vi "Manual Assembly DB.vi"() -> ()   [LabVIEW 2021]
uses:
  Classes/Routine/Routine Enum.ctl
  Classes/Assembly/Database Entry/Database Entry.lvclass
  Classes/Assembly/Assembly Run.lvclass
  Classes/Workspace/Fixture Enum.ctl
  <vilib>/Utility/file.llb/Read Delimited Spreadsheet (string).vi
  SubVIs/PUT_region.vi
  SubVIs/component_tray_region.vi
  SubVIs/assembly_tray_region.vi
  Classes/Controller/I-O/I-O.lvclass
  Classes/Routine/Routine.lvclass
  Classes/Workspace/Fixture.lvclass
  Classes/Controller/Controller.lvclass
panel:
  out "Dummy assembly":bool
  in  "Do old-style single-module data-entry?":bool
  in  "Update comments":bool
  out "Status":string
  out "Stack names":T1
  out "Feet check":bool
  out "Assembly Type":string
  out "Assembly tray region":dbl
  out "Component tray region":dbl
  out "PUT Region":dbl
  in  "Clear All":bool
  in  "Assemble":bool
  in  "Pick and Place":bool
  in  "Dispense glue":bool
  in  "Go":bool
  in  "Routine":T2=enum."Dispense Epoxy"
  in  "Update":bool
  in  "Stage":i32(listbox)=-1
  in  "Stop":bool
  in  "Remove":bool
  in  "Add":bool
  # "Click the Run arrow to start\nFill out pop-up prompts\nSelect Full Assemble\nSelect GO"
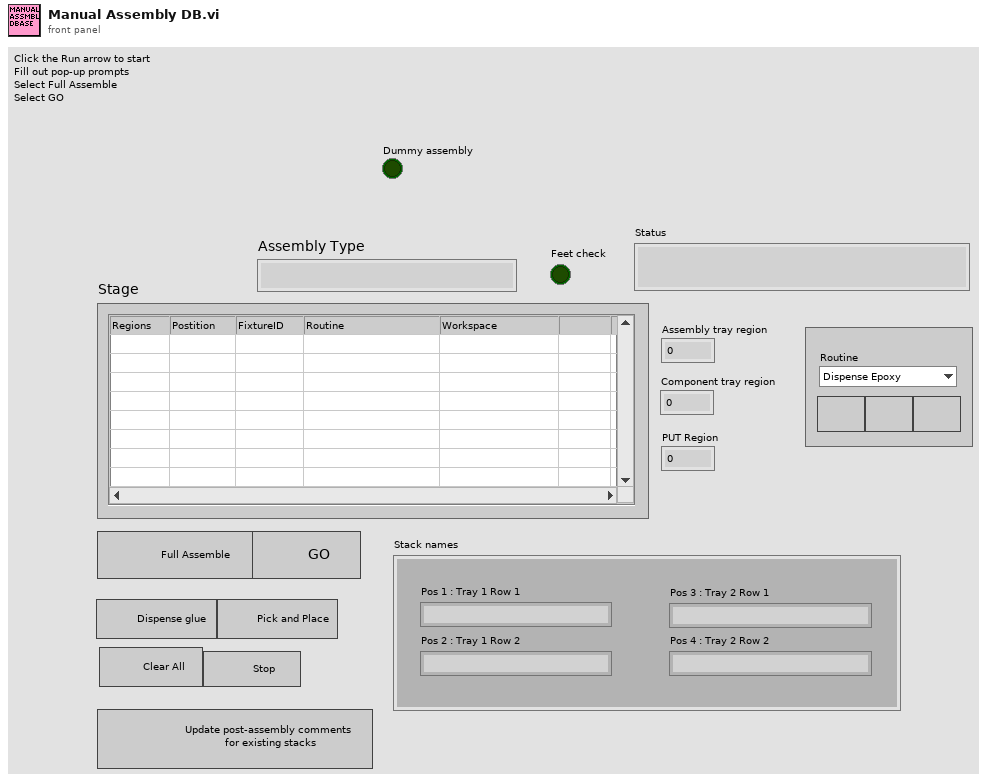
[diagram p1: front panel]
types:
  T1 = cluster{"Pos 1 : Tray 1 Row 1":string, "Pos 2 : Tray 1 Row 2":string, "Pos 3 : Tray 2 Row 1":string, "Pos 4 : Tray 2 Row 2":string}
  T2 = typedef "Routine.lvclass/Routine Enum.ctl" = enum16{"Primary Pick Up", "Secondary Pick Up", "Put Down All", "Secure Syringe", "Release Syringe", "Dispense Epoxy", "Pick Up All", "Put Down Secondary", "Full Assembly"}
  T3 = enum8{"Enabled", "Disabled", "Disabled and Grayed Out"}
  T4 = typedef "Fixture.lvclass/Fixture Enum.ctl" = enum16{"Assembly Tray", "Syringe Space", "Component", "Pick Up Tool", "Current Position"}
  T5 = cluster{"Fixture ID":dbl, "Position":dbl, "Thickness":dbl}
  T6 = typedef "File Paths.ctl" = cluster{"Glue Pattern Folder":path, "Carrier Tray Folder":path, "Pick Up Tool Fixture Folder":path, "Components Folder":path, "Bellows Tool Offset.txt":path, "Pick Up Tool Offset.txt":path, "Dispense Tip Offset.txt":path, "Log Files":path, "Gantry Assembly Map.txt":path, "Syringe and offset map.txt":path, "Controllers Folder":path, "Local dbase config":path}
  T7 = typedef "Controller.lvclass/Controllers.ctl" = cluster{"I-O.lvclass":refnum<class "I-O.lvclass">, "Gantry":refnum<k24>, "Dispenser":refnum<visa-resource-name>}
  T8 = cluster{"Fixture ID":dbl, "Position":dbl, "Thickness":dbl}[]
  T9 = cluster{"Stack names[0]":string, "Stack names[1]":string, "Stack names[2]":string, "Stack names[3]":string}
  T10 = cluster{"Fixture ID":dbl, "Position":dbl, "Thickness":dbl}[][]
  T11 = typedef "I-O.lvclass/Pin Map.ctl" = cluster{"Region Valves":i32[], "Extra Valves":dbl[][][], "Tool Primary Valve":i32, "Tool Secondary Valve":i32, "Region Sensors":i32[], "Extra Sensors":dbl[][][], "Tool Primary Sensor":dbl, "Tool Secondary Sensor":dbl, "Compression Sensor":dbl, "5V":i32, "Dispenser Sensor":dbl}
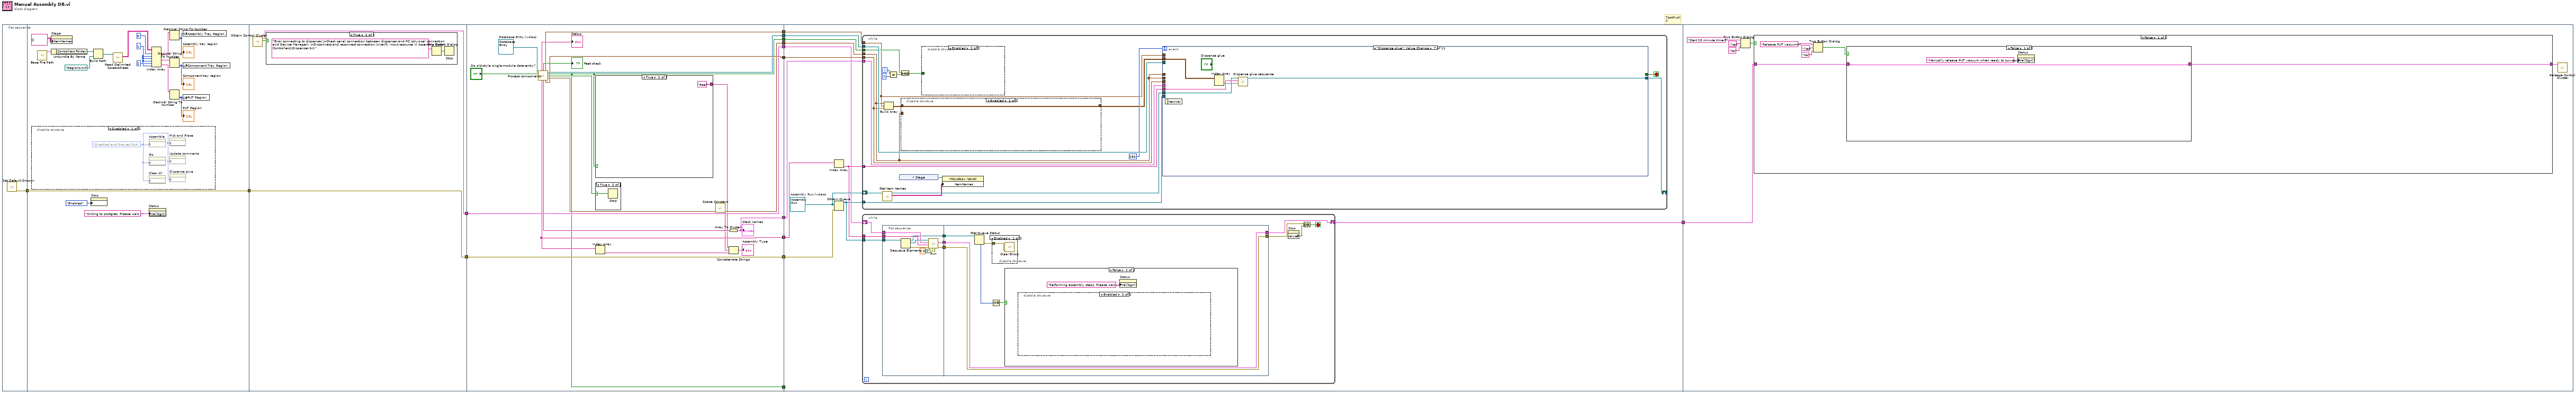
[diagram p0: block diagram]
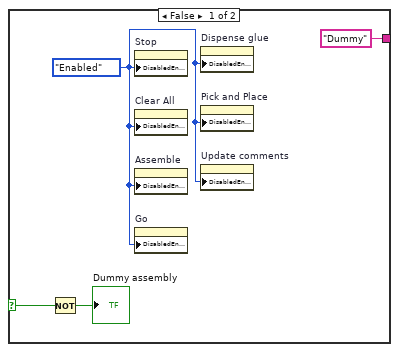
[diagram p4: hidden frame]
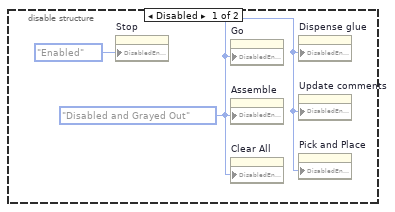
[diagram p7: hidden frame]
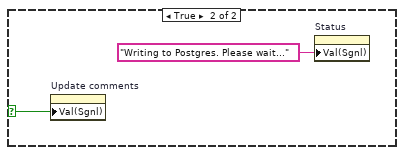
[diagram p8: hidden frame]
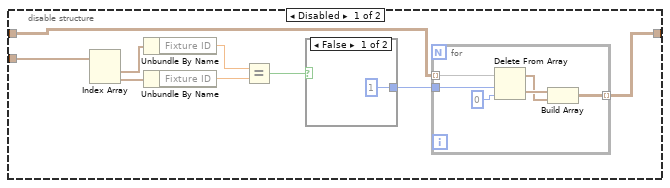
[diagram p9: hidden frame]
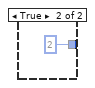
[diagram p10: hidden frame]
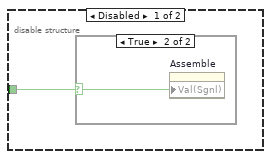
[diagram p11: hidden frame]
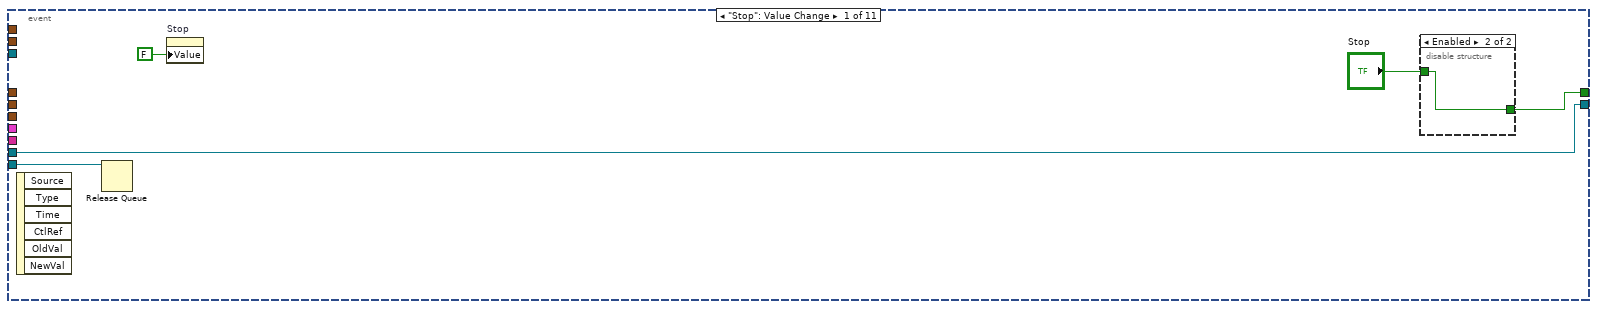
[diagram p13: hidden frame]
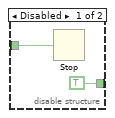
[diagram p14: hidden frame]
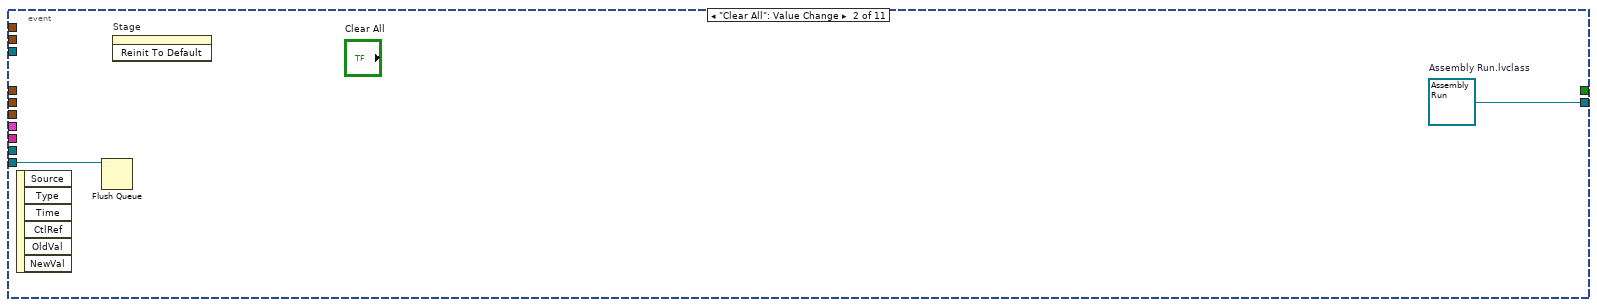
[diagram p15: hidden frame]
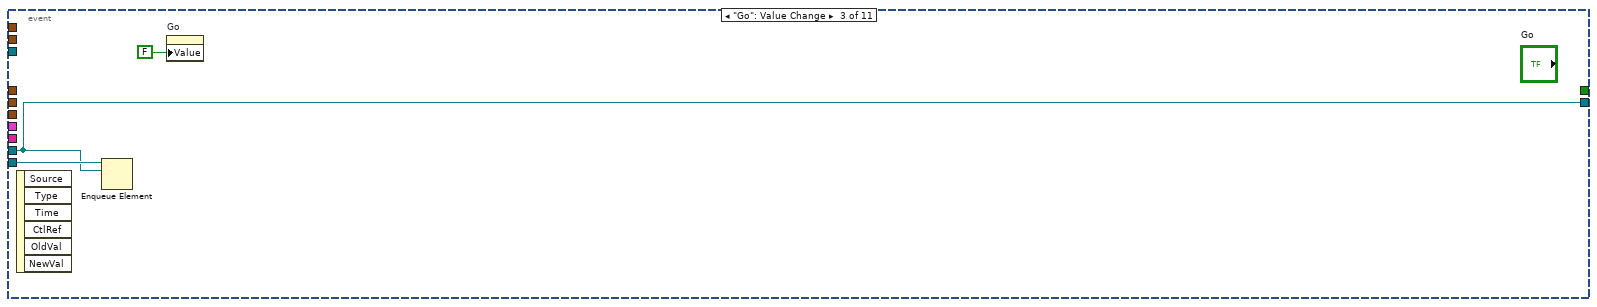
[diagram p16: hidden frame]
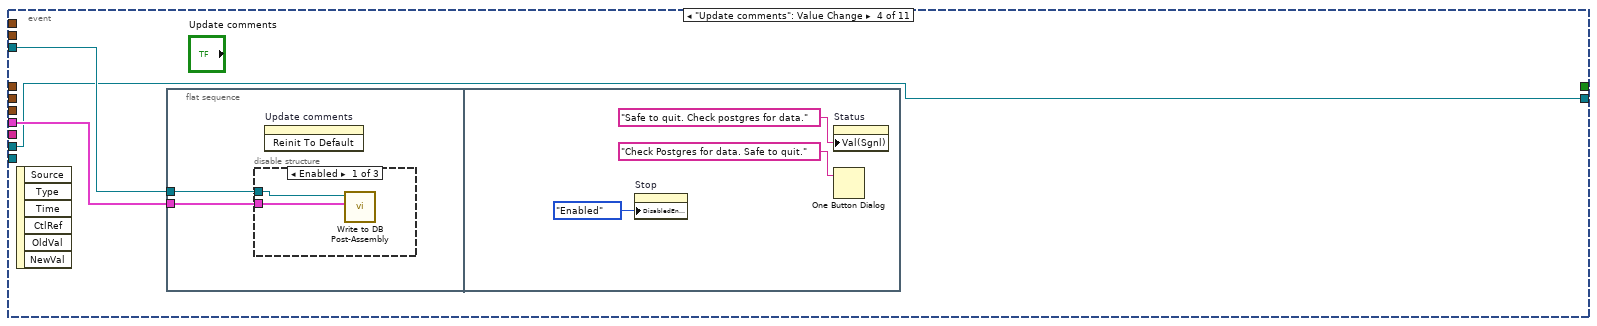
[diagram p17: hidden frame]
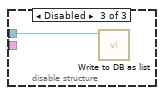
[diagram p19: hidden frame]
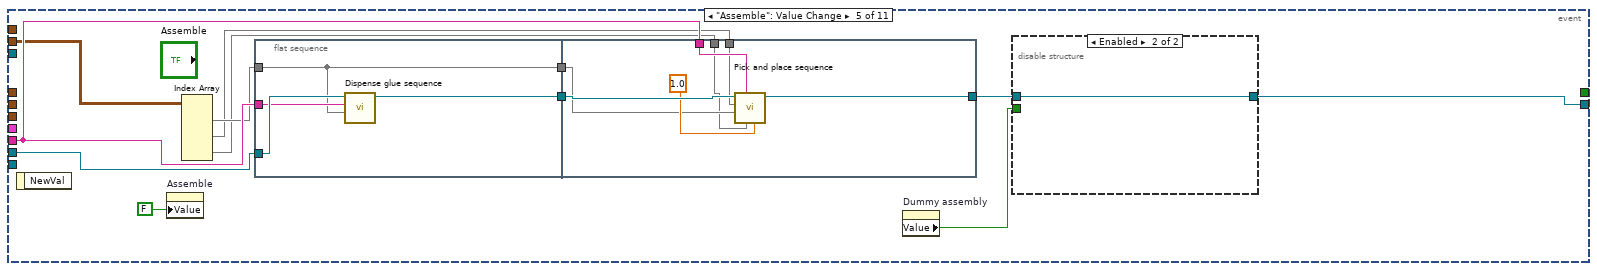
[diagram p20: hidden frame]
diagram:
  # "TestPush\n2"
  n1 = flat-sequence {
    tunnel: [w16] -> w14
    tunnel: [w20] -> w7
    tunnel: w14 -> [w20]
    tunnel: w7 -> [w38]
    tunnel: [w38] -> w6
    tunnel: [w36] -> w4
    tunnel: [w58] -> w15
    tunnel: w6 -> [w58]
    tunnel: [w57] -> w13
    tunnel: [w56] -> w12
    tunnel: [w55] -> w11
    tunnel: [w47] -> w10
    tunnel: [w51] -> w9
    tunnel: [w49] -> w8
    tunnel: [w42] -> w5
    tunnel: w4 -> [w42]
    tunnel: [w41] -> w3
    tunnel: [w41] -> w2
    tunnel: w15 -> [w77]
    tunnel: w13 -> [w76]
    tunnel: w12 -> [w75]
    tunnel: w11 -> [w69]
    tunnel: w10 -> [w74]
    tunnel: w9 -> [w71]
    tunnel: w8 -> [w72]
    tunnel: w5 -> [w68]
    tunnel: w3 -> [w67]
    tunnel: w2 -> [_]
    tunnel: [w66] -> w1
    tunnel: w1 -> [w370]
    frame #0 {
      n2 = call "Set Default Drop-In.vi"() -> ("error out"=w16:errorcluster)  [unwired: 11 in]
    }
    frame #1 {
      w23 = 1 ("disabled index (col)")
      n3 = disable-structure shown="Disabled" {
        frame Disabled {
          w35 = T3."Disabled and Grayed Out" ("Disabled")
          n4 = property on="Assemble" class="Bool (strict)"("DisabledEnum"=w35) -> ()  [unwired: 2 in, 2 out]
          n5 = property on="Go" class="Bool (strict)"("DisabledEnum"=w35) -> ()  [unwired: 2 in, 2 out]
          n6 = property on="Clear All" class="Bool"("DisabledEnum"=w35) -> ()  [unwired: 2 in, 2 out]
          n7 = property on="Pick and Place" class="Bool"("DisabledEnum"=w35) -> ()  [unwired: 2 in, 2 out]
          n8 = property on="Update comments" class="Bool (strict)"("DisabledEnum"=w35) -> ()  [unwired: 2 in, 2 out]
          n9 = property on="Dispense glue" class="Bool"("DisabledEnum"=w35) -> ()  [unwired: 2 in, 2 out]
        }
        frame Enabled {
        }
      }
      n10 = call "Base File Path.vi"() -> ("Paths Out"=w34:T6)  [unwired: 11 in]
      n11 = property on="Stage" class="MCListbox (strict)"("ItemNames"=string[][] []) -> ()  [unwired: 2 in, 2 out]
      n12 = Unbundle By Name(w34) -> ("Controllers Folder"=w32:path)
      n13 = property on="Stop" class="Bool (strict)"("DisabledEnum"=T3."Enabled" ("Disabled")) -> ()  [unwired: 2 in, 2 out]
      n14 = Build Path(base path=w32, name or relative path=path "Regions.txt") -> (appended path=w33:path)
      n15 = call-poly <vilib>:"Read Delimited Spreadsheet.vi"("file path (dialog if empty)"=w33) -> ("all rows"=w21:string[][])  [unwired: 9 in, 5 out]
      n16 = property on="Status" class="Str"("Val(Sgnl)"="Writing to postgres. Please wait..." ("Value (Signaling)")) -> ()  [unwired: 2 in, 2 out]
      n17 = Index Array(array=w21, index (row) #1=0 ("index (row)"), index (col) #1=w23, index (row) #2=w23, index (col) #2=w23, index (row) #3=2 ("disabled index (row)"), index (col) #3=w23) -> (element #1=w26:string, element #2=w25:string, element #3=w27:string)
      n18 = Decimal String To Number(string=w26) -> (number=w29:i32)  [unwired: 2 in, 1 out]
      "Assembly tray region" <- w29
      n19 = Decimal String To Number(string=w25) -> (number=w30:i32)  [unwired: 2 in, 1 out]
      "Component tray region" <- w30
      n20 = Decimal String To Number(string=w27) -> (number=w28:i32)  [unwired: 2 in, 1 out]
      "PUT Region" <- w28
      n21 = global write "assembly_tray_region.vi" "Assembly Tray Region"(w29) -> ()
      n22 = global write "component_tray_region.vi" "Component Tray Region"(w30) -> ()
      n23 = global write "PUT_region.vi" "PUT Region"(w28) -> ()
    }
    frame #2 {
      n24 = call "Obtain Control Cluster.vi"() -> ("Dispenser error?"=w37:bool, "Control Out"=w36:T7)  [unwired: 10 in]
      n25 = case shown="True" w37 {
        frame False {
        }
        frame True {
          n26 = One Button Dialog(message="Error connecting to dispenser.\nCheck serial connection between dispenser and PC (physical connection and Device Manager). \nDisconnect and reconnect connection.\nVerify input resource in Assembly Data\\Controllers\\Dispenser.txt.") -> (true=w39:bool)  [unwired: 1 in]
          n27 = Stop(stop? (T)=w39) -> ()
        }
      }
    }
    frame #3 {
      w59 = refnum<class "Database Entry.lvclass"> refnum  # Database Entry.lvclass
      n28 = call "Process components.vi"("Database Entry in"=w59, "Do single-module data entry?"="Do old-style single-module data-entry?") -> ("Status"=→"Status":string, "Feet check"=→"Feet check":bool, "PUT Settings"=w56:T8, "Database Entry out"=w49:refnum<class "Database Entry.lvclass">, "Is real run?"=w41:bool, "Aborted"=w52:bool, "Assembly Settings"=w55:T8, "Assembly Type"=w47:string[], "Stack names"=w54:string[], "Component Settings"=w57:T8)  [unwired: 3 in, 1 out]
      n29 = case shown="True" w41 {
        selector: w41 -> [w61 _]
        tunnel: ["Dummy" "Real"] -> w44
        frame False {
          w62 = T3."Enabled" ("Disabled")
          n30 = Not(x=w61) -> (.not. x?=→"Dummy assembly":bool)
          n31 = property on="Stop" class="Bool (strict)"("DisabledEnum"=w62) -> ()  [unwired: 2 in, 2 out]
          n32 = property on="Clear All" class="Bool"("DisabledEnum"=w62) -> ()  [unwired: 2 in, 2 out]
          n33 = property on="Assemble" class="Bool (strict)"("DisabledEnum"=w62) -> ()  [unwired: 2 in, 2 out]
          n34 = property on="Go" class="Bool (strict)"("DisabledEnum"=w62) -> ()  [unwired: 2 in, 2 out]
          n35 = property on="Dispense glue" class="Bool"("DisabledEnum"=w62) -> ()  [unwired: 2 in, 2 out]
          n36 = property on="Pick and Place" class="Bool"("DisabledEnum"=w62) -> ()  [unwired: 2 in, 2 out]
          n37 = property on="Update comments" class="Bool (strict)"("DisabledEnum"=w62) -> ()  [unwired: 2 in, 2 out]
        }
        frame True {
        }
      }
      n38 = case shown="True" w52 {
        selector: w52 -> [_ w65]
        frame False {
        }
        frame True {
          n39 = Stop(stop? (T)=w65) -> ()
        }
      }
      n40 = Index Array(array=w47) -> (element=w46:string)  [unwired: 1 in]
      n41 = call <vilib>:"Space Constant.vi"() -> ("String"=w45:string)
      n42 = Array To Cluster(array=w54) -> (cluster=w51:T9)
      "Stack names" <- w51
      n43 = Concatenate Strings(w44, w45, w46) -> (→"Assembly Type":string)
    }
    frame #4 {
      w78 = refnum<class "Assembly Run.lvclass"> refnum  # Assembly Run.lvclass
      n44 = Index Array(array=w74) -> (element=w73:string)  [unwired: 1 in]
      n45 = Obtain Queue(element data type=w78, error in (no error)=w77) -> (queue out=w70:refnum<queue>)  [unwired: 3 in, 2 out]
      n46 = while {
        shift-right: [w125] -> _
        shift-left: w78 -> [w127]
        tunnel: w70 -> [w130]
        tunnel: w73 -> [w124]
        tunnel: w72 -> [w123]
        tunnel: w71 -> [w122]
        tunnel: w75 -> [w114]
        tunnel: w69 -> [w115]
        tunnel: w76 -> [w113]
        tunnel: w67 -> [w121]
        i -> [w120]
        stop <- w131 stop-if-true
        n47 = call "Get Item Names.vi"("Assembly Run in"=w127) -> ("Item names"=w129:string[][], "Assembly Run out"=w126:refnum<class "Assembly Run.lvclass">)  [unwired: 8 in, 1 out]
        n48 = Build Array(w115, w114, w113) -> (w112:T10)
        n49 = Equal?(x=w120, y=1) -> (x = y?=w118:bool)
        n50 = control-ref of="Stage"() -> (w128:refnum<vi>)
        n51 = And(x=w121, y=w118) -> (x .and. y?=w117:bool)
        n52 = disable-structure shown="Enabled" {
          disable-tunnel: w115 -> [w140 _]
          disable-tunnel: w112 -> [w133 w149]
          disable-tunnel: [w132 w149] -> w111
          frame Disabled {
            n53 = Index Array(array=w140) -> (element #1=w139:T5, element #2=w138:T5)  [unwired: 2 in]
            n54 = Unbundle By Name(w139) -> ("Fixture ID"=w137:dbl)
            n55 = Unbundle By Name(w138) -> ("Fixture ID"=w136:dbl)
            n56 = Equal?(x=w137, y=w136) -> (x = y?=w135:bool)
            n57 = case shown="False" w135 {
              tunnel: [1 2] -> w134
              frame False {
              }
              frame True {
              }
            }
            n58 = for {
              tunnel: w133 -> [w146] mode=indexing
              tunnel: [w145] -> w132 mode=indexing
              tunnel: w134 -> [w141]
              n59 = Delete From Array(array=w146, length=w141, index=0) -> (deleted portion=w143:T8, array with subset deleted=w142:T8)
              n60 = Build Array(w143, w142) -> (w145:T10)
            }
          }
          frame Enabled {
          }
        }
        n61 = disable-structure shown="Enabled" {
          disable-tunnel: w117 -> [w150 _]
          frame Disabled {
            n62 = case shown="True" w150 {
              selector: w150 -> [_ w151]
              frame False {
              }
              frame True {
                n63 = property on="Assemble" class="Bool (strict)"("Val(Sgnl)"=w151) -> ()  [unwired: 2 in, 2 out]
              }
            }
          }
          frame Enabled {
          }
        }
        n64 = property class="MCListbox (strict)"(reference=w128, "ItemNames"=w129) -> ()  [unwired: 1 in, 2 out]
        n65 = event shown="[6] \"Dispense glue\": Value Change" {
          selector: _ -> [_ _ _ _ _ _ _ _ _ _ _]
          dyn-events: _ -> [_ _ _ _ _ _ _ _ _ _ _]
          timeout: 250 -> [_ _ _ _ _ _ _ _ _ _ _]
          tunnel: [w153 _ _ _ _ _ _ _ _ _ _] -> w131
          tunnel: w126 -> [w156 _ w163 w165 w187 w206 w211 w219 w229 w361 w364]
          tunnel: [w156 w161 w163 w165 w179 w206 w210 w218 w230 w360 w363] -> w125
          tunnel: w130 -> [w155 w160 w164 _ _ _ _ _ _ _ _]
          tunnel: w113 -> [_ _ _ _ _ _ _ _ _ _ _]
          tunnel: w114 -> [_ _ _ _ _ _ _ _ _ _ _]
          tunnel: w124 -> [_ _ _ _ w186 _ w209 w217 w228 w357 _]
          tunnel: w123 -> [_ _ _ w167 _ _ _ _ _ _ _]
          tunnel: w122 -> [_ _ _ w166 _ _ _ _ _ _ _]
          tunnel: w115 -> [_ _ _ _ _ _ _ _ _ _ _]
          tunnel: w115 -> [_ _ _ _ _ _ _ _ w220 w355 _]
          tunnel: w111 -> [_ _ _ _ w178 _ w208 w212 _ _ _]
          event "Stop": Value Change {
            n66 = event-data() -> ()  [unwired: 1 in, 6 out]
            n67 = Release Queue(queue=w155) -> ()  [unwired: 2 in, 3 out]
            n68 = property on="Stop" class="Bool (strict)"("Value"=FALSE ("Value (Signaling)")) -> ()  [unwired: 2 in, 2 out]
            n69 = disable-structure shown="Enabled" {
              disable-tunnel: "Stop" -> [w158 w159]
              disable-tunnel: [TRUE w159] -> w153
              frame Disabled {
                n70 = Stop(stop? (T)=w158) -> ()
              }
              frame Enabled {
              }
            }
          }
          event "Clear All": Value Change {
            w161 = refnum<class "Assembly Run.lvclass"> refnum  # Assembly Run.lvclass
            n71 = event-data() -> ()  [unwired: 1 in, 6 out]
            n72 = Flush Queue(queue=w160) -> ()  [unwired: 1 in, 3 out]
            n73 = invoke on="Stage" class="MCListbox (strict)" method="Reinit To Default"() -> ()  [unwired: 3 in, 3 out]
          }
          event "Go": Value Change {
            n74 = event-data() -> ()  [unwired: 1 in, 6 out]
            n75 = Enqueue Element(queue=w164, element=w163) -> ()  [unwired: 2 in, 3 out]
            n76 = property on="Go" class="Bool (strict)"("Value"=FALSE ("Go")) -> ()  [unwired: 2 in, 2 out]
          }
          event "Update comments": Value Change {
            n77 = event-data() -> ()  [unwired: 1 in, 6 out]
            n78 = flat-sequence {
              tunnel: w167 -> [w169]
              tunnel: w166 -> [w168]
              frame #0 {
                n79 = disable-structure shown="Enabled" {
                  disable-tunnel: w169 -> [w171 _ w172]
                  disable-tunnel: w168 -> [w170 _ _]
                  frame Enabled {
                    n80 = call "Write to DB Post-Assembly.vi"("Stack names"=w170, "Database Entry in"=w171) -> ()  [unwired: 8 in, 2 out]
                  }
                  frame Disabled {
                  }
                  frame Disabled {
                    n81 = call "Write to DB as list.vi"("Database Entry in"=w172) -> ()  [unwired: 8 in, 3 out]
                  }
                }
                n82 = invoke on="Update comments" class="Bool (strict)" method="Reinit To Default"() -> ()  [unwired: 3 in, 3 out]
              }
              frame #1 {
                n83 = property on="Stop" class="Bool (strict)"("DisabledEnum"=T3."Enabled" ("Disabled")) -> ()  [unwired: 2 in, 2 out]
                n84 = property on="Status" class="Str"("Val(Sgnl)"="Safe to quit. Check postgres for data.") -> ()  [unwired: 2 in, 2 out]
                n85 = One Button Dialog(message="Check Postgres for data. Safe to quit.") -> ()  [unwired: 1 in, 1 out]
              }
            }
          }
          event "Assemble": Value Change {
            n86 = event-data() -> ()  [unwired: 1 in, 1 out]
            n87 = property on="Assemble" class="Bool (strict)"("Value"=FALSE ("Assemble")) -> ()  [unwired: 2 in, 2 out]
            n88 = Index Array(array=w178) -> (element #1=w185:T8, element #2=w184:T8, element #3=w183:T8)  [unwired: 6 in]
            n89 = flat-sequence {
              tunnel: [w190] -> w177
              tunnel: w187 -> [w191]
              tunnel: w186 -> [w189]
              tunnel: w185 -> [w188]
              tunnel: [w188] -> w176
              tunnel: [w197] -> w180
              tunnel: w177 -> [w198]
              tunnel: w186 -> [w196]
              tunnel: w176 -> [w194]
              tunnel: w184 -> [w193]
              tunnel: w183 -> [w192]
              frame #0 {
                n90 = call "Dispense glue sequence.vi"("Assembly Tray Settings Array"=w188, "Assembly Type"=w189, "Assembly Run in"=w191) -> ("Assembly Run out"=w190:refnum<class "Assembly Run.lvclass">)  [unwired: 7 in, 1 out]
              }
              frame #1 {
                n91 = call "Pick and place sequence.vi"("Numeric"=1.0, "Component Tray map"=w192, "Assembly Type"=w196, "Assembly Tray map"=w194, "PUT map"=w193, "Assembly Run in"=w198) -> ("Assembly Run out"=w197:refnum<class "Assembly Run.lvclass">)  [unwired: 4 in, 1 out]
              }
            }
            n92 = property on="Dummy assembly" class="Bool (strict)"() -> ("Value"=w181:bool)  [unwired: 2 in, 2 out]
            n93 = disable-structure shown="Enabled" {
              disable-tunnel: w181 -> [w201 _]
              disable-tunnel: w180 -> [w200 w205]
              disable-tunnel: [w199 w205] -> w179
              frame Disabled {
                n94 = case shown="False" w201 {
                  tunnel: w200 -> [w203 w204]
                  tunnel: [w203 w204] -> w199
                  frame False {
                    n95 = property on="Go" class="Bool (strict)"("Val(Sgnl)"=TRUE ("Value (Signaling)")) -> ()  [unwired: 2 in, 2 out]
                  }
                  frame True {
                  }
                }
              }
              frame Enabled {
              }
            }
          }
          event Timeout {
            n96 = event-data() -> ()  [unwired: 1 in, 3 out]
          }
          event "Dispense glue": Value Change {
            n97 = event-data() -> ()  [unwired: 1 in, 1 out]
            n98 = Index Array(array=w208) -> (element=w207:T8)  [unwired: 2 in]
            n99 = call "Dispense glue sequence.vi"("Assembly Tray Settings Array"=w207, "Assembly Type"=w209, "Assembly Run in"=w211) -> ("Assembly Run out"=w210:refnum<class "Assembly Run.lvclass">)  [unwired: 7 in, 1 out]
          }
          event "Pick and Place": Value Change {
            n100 = event-data() -> ()  [unwired: 1 in, 6 out]
            n101 = Index Array(array=w212) -> (element #1=w215:T8, element #2=w214:T8, element #3=w213:T8)  [unwired: 6 in]
            n102 = call "Pick and place sequence.vi"("Numeric"=1.0, "Component Tray map"=w213, "Assembly Type"=w217, "Assembly Tray map"=w215, "PUT map"=w214, "Assembly Run in"=w219) -> ("Assembly Run out"=w218:refnum<class "Assembly Run.lvclass">)  [unwired: 4 in, 1 out]
          }
          event "Add": Value Change {
            n103 = event-data() -> ()  [unwired: 1 in, 1 out]
            n104 = local read "Routine"() -> (w224:T2)
            n105 = case shown="\"Primary Pick Up\"" w224 {
              tunnel: [Fixture_Enum."Assembly Tray" ("Fixture") Fixture_Enum."Pick Up Tool" ("Fixture") Fixture_Enum."Component" ("Fixture") Fixture_Enum."Assembly Tray" ("Fixture") Fixture_Enum."Assembly Tray" ("Fixture") Fixture_Enum."Assembly Tray" ("Fixture") Fixture_Enum."Syringe Space" ("Fixture") Fixture_Enum."Syringe Space" ("Fixture")] -> w227
              tunnel: w220 -> [w252 w255 w274 w293 w312 w331 w350 w353]
              tunnel: [_ w254 w275 w292 w311 w330 w349 w352] -> w221
              tunnel: [w252 _ _ _ _ _ _ _] -> w222
              frame "Dispense Epoxy", Default {
              }
              frame "Primary Pick Up" {
                n106 = call "Prompt User for Input"() -> ("Position"=w256:dbl)  [unwired: 17 in, 2 out]
                n107 = for {
                  tunnel: w256 -> [w258]
                  tunnel: w255 -> [w262] mode=indexing
                  tunnel: [w259] -> w254
                  stop <- w260 stop-if-true
                  n108 = Unbundle By Name(w262) -> ("Position"=w263:dbl)
                  n109 = Equal?(x=w263, y=w258) -> (x = y?=w261:bool)
                  n110 = case shown="False" w261 {
                    selector: w261 -> [w270 w272]
                    tunnel: w262 -> [_ w271]
                    tunnel: [w270 w272] -> w260
                    tunnel: [T5 {"Fixture ID"=0.0, "Position"=0.0, "Thickness"=0.0} ("Settings") w271] -> w259
                    tunnel: w258 -> [w265 _]
                    frame False {
                      n111 = Number To Decimal String(number=w265) -> (decimal integer string=w266:string)  [unwired: 1 in]
                      n112 = Concatenate Strings("Position " ("message"), w266, " not available." ("message")) -> (w264:string)
                      n113 = One Button Dialog(message=w264) -> ()  [unwired: 1 in, 1 out]
                    }
                    frame True {
                    }
                  }
                }
              }
              frame "Secondary Pick Up" {
                n114 = call "Prompt User for Input2"() -> ("Position"=w273:dbl)  [unwired: 17 in, 2 out]
                n115 = for {
                  tunnel: w273 -> [w277]
                  tunnel: w274 -> [w281] mode=indexing
                  tunnel: [w278] -> w275
                  stop <- w279 stop-if-true
                  n116 = Unbundle By Name(w281) -> ("Position"=w282:dbl)
                  n117 = Equal?(x=w282, y=w277) -> (x = y?=w280:bool)
                  n118 = case shown="False" w280 {
                    selector: w280 -> [w289 w291]
                    tunnel: w281 -> [_ w290]
                    tunnel: [w289 w291] -> w279
                    tunnel: [T5 {"Fixture ID"=0.0, "Position"=0.0, "Thickness"=0.0} ("Settings") w290] -> w278
                    tunnel: w277 -> [w284 _]
                    frame False {
                      n119 = Number To Decimal String(number=w284) -> (decimal integer string=w285:string)  [unwired: 1 in]
                      n120 = Concatenate Strings("Position " ("message"), w285, " not available." ("message")) -> (w283:string)
                      n121 = One Button Dialog(message=w283) -> ()  [unwired: 1 in, 1 out]
                    }
                    frame True {
                    }
                  }
                }
              }
              frame "Pick Up All" {
                n122 = call "Prompt User for Input3"() -> ("Position"=w294:dbl)  [unwired: 17 in, 2 out]
                n123 = for {
                  tunnel: w294 -> [w296]
                  tunnel: w293 -> [w300] mode=indexing
                  tunnel: [w297] -> w292
                  stop <- w298 stop-if-true
                  n124 = Unbundle By Name(w300) -> ("Position"=w301:dbl)
                  n125 = Equal?(x=w301, y=w296) -> (x = y?=w299:bool)
                  n126 = case shown="False" w299 {
                    selector: w299 -> [w308 w310]
                    tunnel: w300 -> [_ w309]
                    tunnel: [w308 w310] -> w298
                    tunnel: [T5 {"Fixture ID"=0.0, "Position"=0.0, "Thickness"=0.0} ("Settings") w309] -> w297
                    tunnel: w296 -> [w303 _]
                    frame False {
                      n127 = Number To Decimal String(number=w303) -> (decimal integer string=w304:string)  [unwired: 1 in]
                      n128 = Concatenate Strings("Position " ("message"), w304, " not available." ("message")) -> (w302:string)
                      n129 = One Button Dialog(message=w302) -> ()  [unwired: 1 in, 1 out]
                    }
                    frame True {
                    }
                  }
                }
              }
              frame "Put Down Secondary" {
                n130 = call "Prompt User for Input4"() -> ("Position"=w313:dbl)  [unwired: 17 in, 2 out]
                n131 = for {
                  tunnel: w313 -> [w315]
                  tunnel: w312 -> [w319] mode=indexing
                  tunnel: [w316] -> w311
                  stop <- w317 stop-if-true
                  n132 = Unbundle By Name(w319) -> ("Position"=w320:dbl)
                  n133 = Equal?(x=w320, y=w315) -> (x = y?=w318:bool)
                  n134 = case shown="False" w318 {
                    selector: w318 -> [w327 w329]
                    tunnel: w319 -> [_ w328]
                    tunnel: [w327 w329] -> w317
                    tunnel: [T5 {"Fixture ID"=0.0, "Position"=0.0, "Thickness"=0.0} ("Settings") w328] -> w316
                    tunnel: w315 -> [w322 _]
                    frame False {
                      n135 = Number To Decimal String(number=w322) -> (decimal integer string=w323:string)  [unwired: 1 in]
                      n136 = Concatenate Strings("Position " ("message"), w323, " not available." ("message")) -> (w321:string)
                      n137 = One Button Dialog(message=w321) -> ()  [unwired: 1 in, 1 out]
                    }
                    frame True {
                    }
                  }
                }
              }
              frame "Put Down All" {
                n138 = call "Prompt User for Input5"() -> ("Position"=w332:dbl)  [unwired: 17 in, 2 out]
                n139 = for {
                  tunnel: w332 -> [w334]
                  tunnel: w331 -> [w338] mode=indexing
                  tunnel: [w335] -> w330
                  stop <- w336 stop-if-true
                  n140 = Unbundle By Name(w338) -> ("Position"=w339:dbl)
                  n141 = Equal?(x=w339, y=w334) -> (x = y?=w337:bool)
                  n142 = case shown="False" w337 {
                    selector: w337 -> [w346 w348]
                    tunnel: w338 -> [_ w347]
                    tunnel: [w346 w348] -> w336
                    tunnel: [T5 {"Fixture ID"=0.0, "Position"=0.0, "Thickness"=0.0} ("Settings") w347] -> w335
                    tunnel: w334 -> [w341 _]
                    frame False {
                      n143 = Number To Decimal String(number=w341) -> (decimal integer string=w342:string)  [unwired: 1 in]
                      n144 = Concatenate Strings("Position " ("message"), w342, " not available." ("message")) -> (w340:string)
                      n145 = One Button Dialog(message=w340) -> ()  [unwired: 1 in, 1 out]
                    }
                    frame True {
                    }
                  }
                }
              }
              frame "Secure Syringe" {
                n146 = Index Array(array=w350) -> (element=w349:T5)  [unwired: 1 in]
              }
              frame "Release Syringe" {
                n147 = Index Array(array=w353) -> (element=w352:T5)  [unwired: 1 in]
              }
            }
            n148 = Equal?(x=w224, y=Routine_Enum."Dispense Epoxy") -> (x = y?=w225:bool)
            n149 = case shown="True" w225 {
              tunnel: [w237 w251] -> w230
              tunnel: w229 -> [w236 w250]
              tunnel: w228 -> [w235 w249]
              tunnel: w227 -> [w234 w248]
              tunnel: w224 -> [w233 w247]
              tunnel: TRUE ("Auto") -> [w232 w246]
              tunnel: w222 -> [w231 _]
              tunnel: w221 -> [_ w245]
              frame True {
                n150 = for {
                  tunnel: w235 -> [w242]
                  tunnel: w234 -> [w241]
                  tunnel: w233 -> [w240]
                  tunnel: w232 -> [w239]
                  shift-right: [w244] -> w237
                  shift-left: w236 -> [w243]
                  tunnel: w231 -> [w238] mode=indexing
                  n151 = call-dynamic "Add Single.vi"("UI in"=w243, "Routine"=w240, "Assembly Type"=w242, "Fixture"=w241, "Input Settings"=w238, "Auto"=w239) -> ("UI out"=w244:refnum<class "Assembly Run.lvclass">)  [unwired: 8 in, 1 out]
                }
              }
              frame False {
                n152 = call-dynamic "Add Single.vi"("UI in"=w250, "Routine"=w247, "Assembly Type"=w249, "Fixture"=w248, "Input Settings"=w245, "Auto"=w246) -> ("UI out"=w251:refnum<class "Assembly Run.lvclass">)  [unwired: 8 in, 1 out]
              }
            }
          }
          event "Update": Value Change {
            n153 = event-data() -> ()  [unwired: 1 in, 6 out]
            n154 = Index Array(array=w355) -> (element=w356:T5)  [unwired: 1 in]
            n155 = call "Update.vi"("Input Settings"=w356, "Assembly Type"=w357, "Row"="Stage", "Routine"="Routine", "Assembly Run in"=w361) -> ("Assembly Run out"=w360:refnum<class "Assembly Run.lvclass">)  [unwired: 5 in, 1 out]
          }
          event "Remove": Value Change {
            n156 = event-data() -> ()  [unwired: 1 in, 6 out]
            n157 = local read "Stage"() -> (w362:i32)
            n158 = call "Delete.vi"("Index"=w362, "Assembly In"=w364) -> ("Assembly Out"=w363:refnum<class "Assembly Run.lvclass">)  [unwired: 8 in, 1 out]
          }
        }
      }
      n159 = while {
        shift-right: [w87] -> w66
        shift-left: w68 -> [w88]
        tunnel: w73 -> [w86]
        tunnel: w70 -> [w85]
        stop <- w80 stop-if-true
        n160 = flat-sequence {
          tunnel: w88 -> [w96]
          tunnel: w86 -> [w94]
          tunnel: w85 -> [w91]
          tunnel: [w95] -> w84
          tunnel: [w93] -> w83
          tunnel: [w92] -> w82
          tunnel: [w103] -> w81
          tunnel: [w104] -> w87
          tunnel: w84 -> [w104]
          tunnel: w83 -> [w103]
          tunnel: w82 -> [w102]
          frame #0 {
            n161 = Dequeue Element(queue=w91) -> (queue out=w92:refnum<queue>, element=w98:refnum<class "Assembly Run.lvclass">, error out=w97:errorcluster)  [unwired: 2 in, 1 out]
            n162 = call-dynamic "Run.vi"("Dispense?"=TRUE, "Pickup_Test_Number"=0.0, "error in (no error)"=w97, "Assembly Type"=w94, "Control In"=w96, "Assembly In"=w98) -> ("error out"=w93:errorcluster, "Control Out"=w95:T7)  [unwired: 3 in, 1 out]
          }
          frame #1 {
            n163 = Get Queue Status(queue=w102) -> (error out=w99:errorcluster, # elements in queue=w101:i32)  [unwired: 2 in, 6 out]
            n164 = Equal To 0?(x=w101) -> (x = 0?=w100:bool)
            n165 = disable-structure shown="Enabled" {
              disable-tunnel: w99 -> [w105 _]
              frame Enabled {
                n166 = call <vilib>:"Clear Errors.vi"("error in (no error)"=w105) -> ()  [unwired: 5 in, 2 out]
              }
              frame Disabled {
              }
            }
            n167 = case shown="False" w100 {
              selector: w100 -> [_ w110]
              frame False {
                n168 = disable-structure shown="Enabled" {
                  frame Disabled {
                    w108 = T3."Disabled and Grayed Out" ("Disabled")
                    n169 = property on="Stop" class="Bool (strict)"("DisabledEnum"=T3."Enabled" ("Disabled")) -> ()  [unwired: 2 in, 2 out]
                    n170 = property on="Go" class="Bool (strict)"("DisabledEnum"=w108) -> ()  [unwired: 2 in, 2 out]
                    n171 = property on="Assemble" class="Bool (strict)"("DisabledEnum"=w108) -> ()  [unwired: 2 in, 2 out]
                    n172 = property on="Clear All" class="Bool"("DisabledEnum"=w108) -> ()  [unwired: 2 in, 2 out]
                    n173 = property on="Dispense glue" class="Bool"("DisabledEnum"=w108) -> ()  [unwired: 2 in, 2 out]
                    n174 = property on="Update comments" class="Bool (strict)"("DisabledEnum"=w108) -> ()  [unwired: 2 in, 2 out]
                    n175 = property on="Pick and Place" class="Bool"("DisabledEnum"=w108) -> ()  [unwired: 2 in, 2 out]
                  }
                  frame Enabled {
                  }
                }
                n176 = property on="Status" class="Str"("Val(Sgnl)"="Performing assembly steps. Please wait...") -> ()  [unwired: 2 in, 2 out]
              }
              frame True {
                n177 = property on="Update comments" class="Bool (strict)"("Val(Sgnl)"=w110) -> ()  [unwired: 2 in, 2 out]
                n178 = property on="Status" class="Str"("Val(Sgnl)"="Writing to Postgres. Please wait...") -> ()  [unwired: 2 in, 2 out]
              }
            }
          }
        }
        n179 = property on="Stop" class="Bool (strict)"() -> ("Value"=w79:bool)  [unwired: 2 in, 2 out]
        n180 = Or(x=w81, y=w79) -> (x .or. y?=w80:bool)
      }
    }
    frame #5 {
      n181 = Two Button Dialog(message="Start 20 minute timer?", 1:"No" ("F button name (\"Cancel\")"), 2:"Yes" ("T button name (\"OK\")")) -> (T button?=w365:bool)
      n182 = case shown="False" w365 {
        tunnel: w370 -> [w376 w404]
        tunnel: [w375 w400] -> w369
        frame False {
          n183 = Two Button Dialog(message="Release PUT vacuum?", 1:"No" ("F button name (\"Cancel\")"), 2:"Yes" ("T button name (\"OK\")")) -> (T button?=w371:bool)
          n184 = case shown="False" w371 {
            tunnel: w376 -> [w378 w381]
            tunnel: [w378 w379] -> w375
            frame False {
              n185 = property on="Status" class="Str"("Val(Sgnl)"="Manually release PUT vacuum when ready to survey." ("Value (Signaling)")) -> ()  [unwired: 2 in, 2 out]
            }
            frame True {
              n186 = flat-sequence {
                tunnel: w381 -> [w383]
                tunnel: [w382] -> w380
                tunnel: w380 -> [w398]
                tunnel: [w398] -> w379
                frame #0 {
                  n187 = in-place {
                    n188 = in-place-cluster #1(w383) -> ("I-O.lvclass"=w385:refnum<class "I-O.lvclass">)
                    n189 = call-dynamic "Read Pin Map.vi"("I-O in"=w385) -> ("Pin Map 2"=w390:T11, "I-O out"=w387:refnum<class "I-O.lvclass">)  [unwired: 8 in, 1 out]
                    n190 = Unbundle By Name(w390) -> ("Extra Valves"=w389:dbl[][][])
                    n191 = Index Array(array=w389, index (dim 0)=0 ("index (page)")) -> (element=w388:dbl[][])  [unwired: 2 in]
                    n192 = for {
                      tunnel: w388 -> [w396] mode=indexing
                      shift-right: [w394] -> w384
                      shift-left: w387 -> [w395]
                      n193 = Index Array(array=w396, index=0) -> (element=w393:dbl)
                      n194 = call-dynamic "Digital Write 1 Channel.vi"("Value"=FALSE, "Channel"=w393, "I-O.lvclass"=w395) -> ("I-O.lvclass 2"=w394:refnum<class "I-O.lvclass">)  [unwired: 7 in, 1 out]
                    }
                    n195 = in-place-cluster #1("I-O.lvclass"=w384) -> (w382:T7)
                  }
                }
                frame #1 {
                  n196 = property on="Status" class="Str"("Val(Sgnl)"="PUT vacuum has been released." ("Value (Signaling)")) -> ()  [unwired: 2 in, 2 out]
                }
              }
            }
          }
        }
        frame True {
          n197 = flat-sequence {
            tunnel: w404 -> [w406]
            tunnel: [w405] -> w403
            tunnel: w403 -> [w428]
            tunnel: [w428] -> w402
            tunnel: [w425] -> w401
            tunnel: w402 -> [w430]
            tunnel: w401 -> [w431]
            tunnel: [w429] -> w399
            tunnel: [w454] -> w400
            tunnel: w399 -> [w454]
            frame #0 {
              n198 = while {
                shift-right: [w419] -> w405
                shift-left: w406 -> [w419]
                stop <- w423 stop-if-true
                w413 = "%#g" ("format string")
                w422 = 1200.0 ("Time Target (s)")
                n199 = call "Elapsed Time"("Time Target (s)"=w422) -> ("Elapsed Time (s)"=w421:dbl, "Time has Elapsed"=w423:bool)  [unwired: 11 in, 6 out]
                n200 = Subtract(x=w422, y=w421) -> (x-y=w418:dbl)
                n201 = Quotient & Remainder(x=w418, y=60.0) -> (x-y*floor(x/y)=w416:dbl, floor(x/y)=w415:dbl)
                n202 = Round To Nearest(number=w416) -> (nearest integer value=w408:dbl)
                n203 = Round To Nearest(number=w415) -> (nearest integer value=w407:dbl)
                n204 = Format Into String(format string=w413, initial string="PUT vacuum will release after ", w407) -> (resulting string=w410:string)  [unwired: 1 in, 1 out]
                n205 = Format Into String(format string=w413, initial string=" minutes and ", w408) -> (resulting string=w414:string)  [unwired: 1 in, 1 out]
                n206 = Concatenate Strings(w410, w414, " seconds." ("string")) -> (w417:string)
                n207 = property on="Status" class="Str"("Val(Sgnl)"=w417) -> ()  [unwired: 2 in, 2 out]
              }
            }
            frame #1 {
              n208 = Two Button Dialog(message="20 minute curing period is complete. Release PUT vacuum?", 1:"No" ("F button name (\"Cancel\")"), 2:"Yes" ("T button name (\"OK\")")) -> (T button?=w425:bool)
            }
            frame #2 {
              n209 = case shown="True" w431 {
                tunnel: w430 -> [w433 w436]
                tunnel: [w433 w434] -> w429
                frame False {
                  n210 = property on="Status" class="Str"("Val(Sgnl)"="Manually release PUT vacuum when ready to survey." ("Value (Signaling)")) -> ()  [unwired: 2 in, 2 out]
                }
                frame True {
                  n211 = flat-sequence {
                    tunnel: w436 -> [w438]
                    tunnel: [w437] -> w435
                    tunnel: w435 -> [w453]
                    tunnel: [w453] -> w434
                    frame #0 {
                      n212 = in-place {
                        n213 = in-place-cluster #2(w438) -> ("I-O.lvclass"=w440:refnum<class "I-O.lvclass">)
                        n214 = call-dynamic "Read Pin Map.vi"("I-O in"=w440) -> ("Pin Map 2"=w445:T11, "I-O out"=w442:refnum<class "I-O.lvclass">)  [unwired: 8 in, 1 out]
                        n215 = Unbundle By Name(w445) -> ("Extra Valves"=w444:dbl[][][])
                        n216 = Index Array(array=w444, index (dim 0)=0 ("index (page)")) -> (element=w443:dbl[][])  [unwired: 2 in]
                        n217 = for {
                          tunnel: w443 -> [w451] mode=indexing
                          shift-right: [w449] -> w439
                          shift-left: w442 -> [w450]
                          n218 = Index Array(array=w451, index=0) -> (element=w448:dbl)
                          n219 = call-dynamic "Digital Write 1 Channel.vi"("Value"=FALSE, "Channel"=w448, "I-O.lvclass"=w450) -> ("I-O.lvclass 2"=w449:refnum<class "I-O.lvclass">)  [unwired: 7 in, 1 out]
                        }
                        n220 = in-place-cluster #2("I-O.lvclass"=w439) -> (w437:T7)
                      }
                    }
                    frame #1 {
                      n221 = property on="Status" class="Str"("Val(Sgnl)"="PUT vacuum has been released." ("Value (Signaling)")) -> ()  [unwired: 2 in, 2 out]
                    }
                  }
                }
              }
            }
            frame #3 {
              n222 = disable-structure shown="Enabled" {
                frame Disabled {
                  n223 = property on="Stop" class="Bool (strict)"("Val(Sgnl)"=TRUE ("Value (Signaling)")) -> ()  [unwired: 2 in, 2 out]
                }
                frame Enabled {
                }
              }
            }
          }
        }
      }
      n224 = call "Release Control Cluster.vi"("output cluster"=w369) -> ()  [unwired: 11 in]
    }
  }
